vi "Config.View.vi"() -> ()   [LabVIEW 2019]
uses:
  Telas.ctl
  <vilib>/Utility/miscctls.llb/LVPositionTypeDef.ctl
  <vilib>/Utility/miscctls.llb/LVPointTypeDef.ctl
panel:
  out "ProximaTela":T1
  in  "Tab":enum32{"Page 1", "Page 2"}(tab)
  in  "Voltar":bool
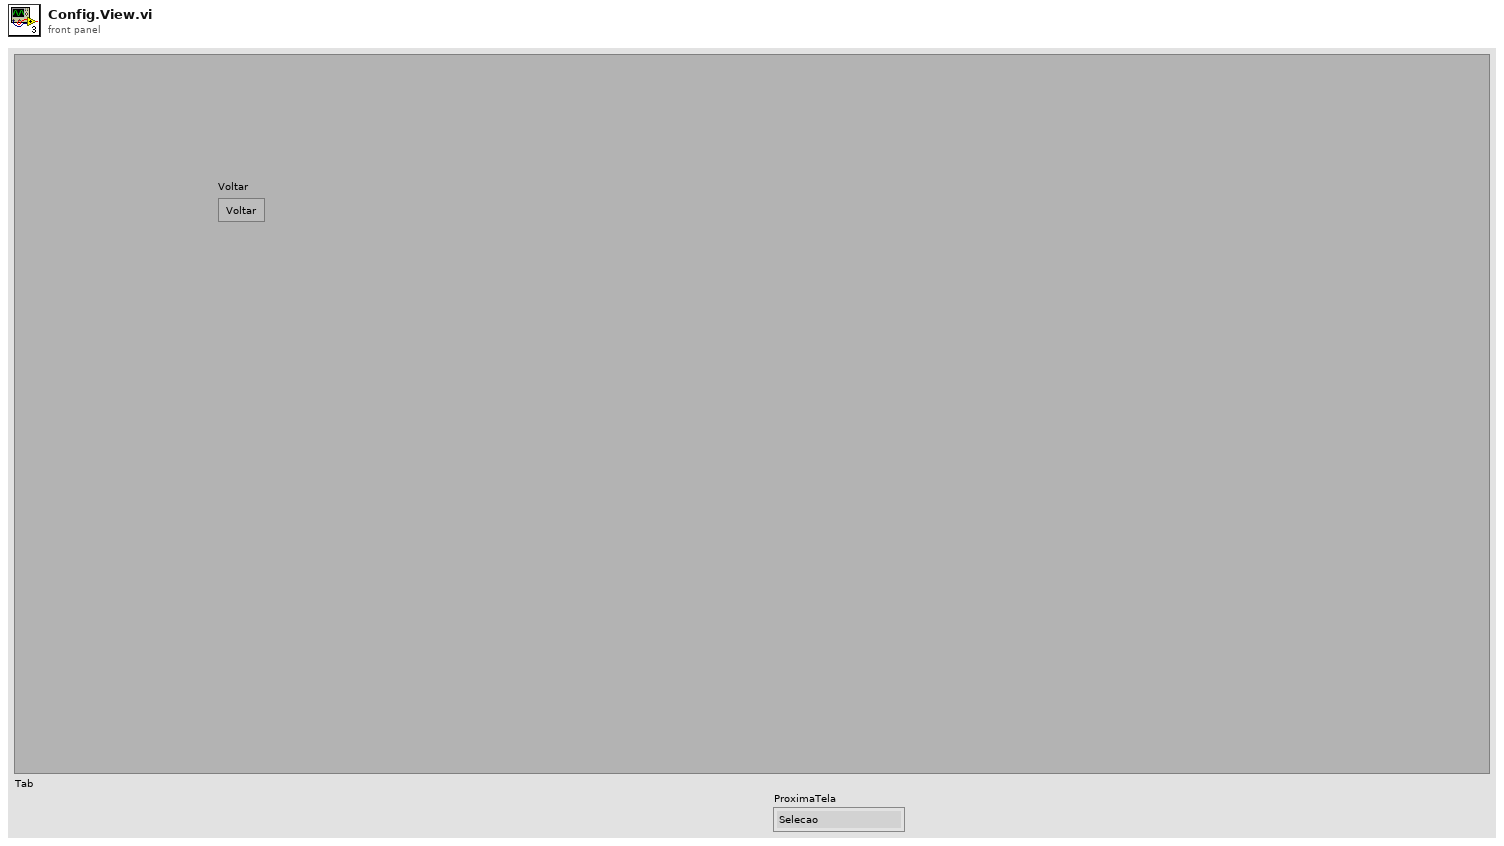
[diagram p1: front panel]
types:
  T1 = typedef "Telas.ctl" = enum16{"Selecao", "Config", "Medicao"}
  T2 = typedef "LVPositionTypeDef.ctl" = cluster{"Left":i32, "Top":i32}
  T3 = typedef "LVPointTypeDef.ctl" = cluster{"Horizontal":i16, "Vertical":i16}
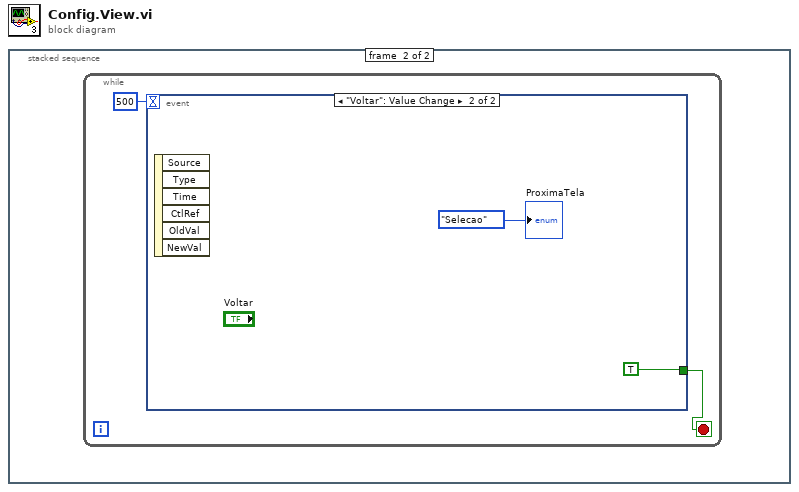
[diagram p0: block diagram]
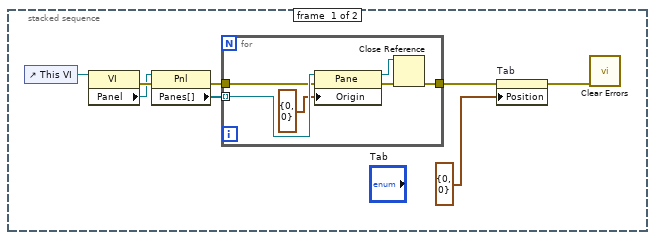
[diagram p2: hidden frame]
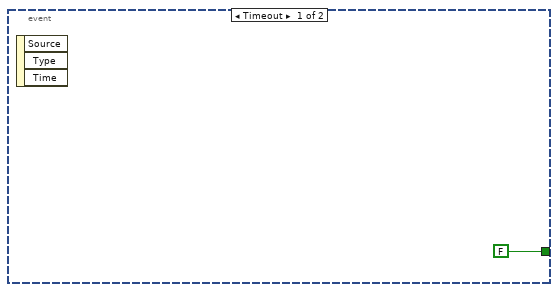
[diagram p3: hidden frame]
diagram:
  n1 = stacked-sequence {
    frame #0 {
      n2 = control-ref of="This VI"() -> (w5:refnum<vi>)
      n3 = property class="VI"(reference=w5) -> (error out=w8:errorcluster, "Panel"=w7:refnum<vi>)  [unwired: 1 in, 1 out]
      n4 = property class="Pnl"(reference=w7, error in=w8) -> (error out=w4:errorcluster, "Panes[]"=w6:refnum<vi>[])  [unwired: 1 out]
      n5 = for {
        tunnel: w6 -> [w14] mode=indexing
        tunnel: w4 -> [w10]
        tunnel: [w9] -> w3
        n6 = property class="Pane"(reference=w14, error in=w10, "Origin"=T3 {"Horizontal"=0, "Vertical"=0}) -> (reference out=w11:refnum<vi>, error out=w12:errorcluster)
        n7 = Close Reference(reference=w11, error in (no error)=w12) -> (error out=w9:errorcluster)
      }
      n8 = property on="Tab" class="TabCtl (strict)"(error in=w3, "Position"=T2 {"Left"=0, "Top"=0}) -> (error out=w2:errorcluster)  [unwired: 1 in, 1 out]
      n9 = call <vilib>:"Clear Errors.vi"("error in (no error)"=w2) -> ()  [unwired: 5 in, 2 out]
    }
    frame #1 {
      n10 = while {
        stop <- w15 stop-if-true
        n11 = event shown="[1] \"Voltar\": Value Change" {
          selector: _ -> [_ _]
          dyn-events: _ -> [_ _]
          timeout: 500 -> [_ _]
          tunnel: [FALSE TRUE] -> w15
          event Timeout {
            n12 = event-data() -> ()  [unwired: 1 in, 3 out]
          }
          event "Voltar": Value Change {
            n13 = event-data() -> ()  [unwired: 1 in, 6 out]
            "ProximaTela" <- Telas."Selecao" ("NextScreen")
          }
        }
      }
    }
  }
